vi "H-Bridge Control.vi"(11 "PWM Value (-2000 to 2000)":i16) -> (2 "PWM B":u16, 3 "PWM A":u16)   [LabVIEW 2018]
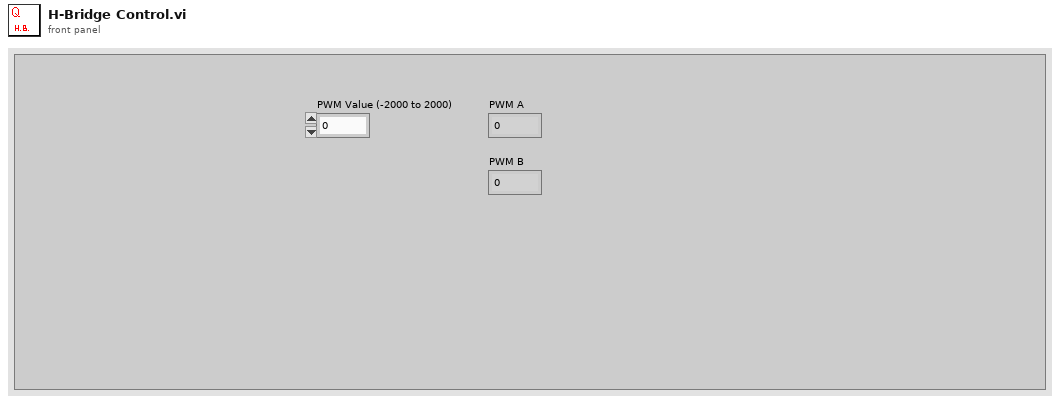
[diagram p1: front panel]
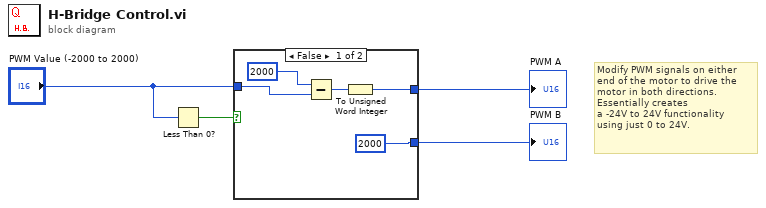
[diagram p0: block diagram]
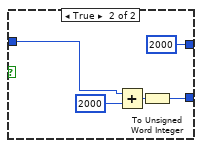
[diagram p2: hidden frame]
diagram:
  # "Modify PWM signals on either\nend of the motor to drive the \nmotor in both directions. \nEssentially creates\na -24V to 24V functionality \nusing just 0 to 24V."
  n1 = Less Than 0?(x="PWM Value (-2000 to 2000)") -> (x < 0?=w1:bool)
  n2 = case shown="False" w1 {
    tunnel: "PWM Value (-2000 to 2000)" -> [w9 w12]
    tunnel: [w5 u16 2000] -> w3
    tunnel: [u16 2000 ("x 3") w10] -> w4
    frame False {
      n3 = Subtract ("Subtract 2")(x=i16 2000, y=w9) -> (x-y=w7:i16)
      n4 = To Unsigned Word Integer ("To Unsigned Word Integer 3")(number=w7) -> (unsigned 16bit integer=w5:u16)
    }
    frame True {
      n5 = Add ("Add 2")(x=w12, y=i16 2000 ("3")) -> (x+y=w11:i16)
      n6 = To Unsigned Word Integer ("To Unsigned Word Integer 4")(number=w11) -> (unsigned 16bit integer=w10:u16)
    }
  }
  "PWM B" <- w4
  "PWM A" <- w3
